vi "svm_save_model.vi"(8 "error in (no error)":errorcluster, 10 "Model":T1, 11 "Save path":path) -> (0 "error out":errorcluster)   [LabVIEW 2015]
uses:
  Controls/svm_model.ctl
  Controls/svm_parameter.ctl
  Controls/svm_type.ctl
  Controls/svm_kernel_type.ctl
  Controls/svm_node.ctl
  bin/LabVIEW-libsvm.so
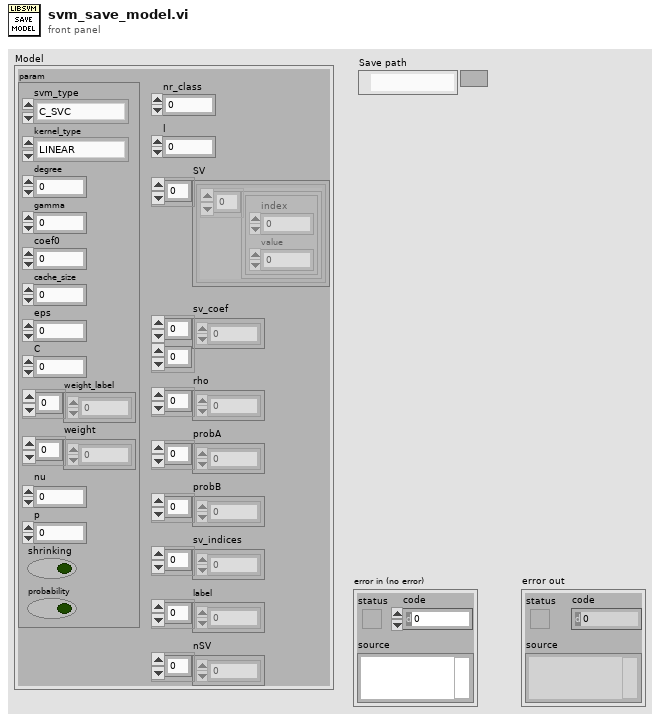
[diagram p1: front panel]
types:
  T1 = typedef "svm_model.ctl" = cluster{"param":T2, "nr_class":i32, "l":i32, "SV":cluster{"Array":T5[]}[], "sv_coef":dbl[][], "rho":dbl[], "probA":dbl[], "probB":dbl[], "sv_indices":i32[], "label":i32[], "nSV":i32[]}
  T2 = typedef "svm_parameter.ctl" = cluster{"svm_type":T3, "kernel_type":T4, "degree":i32, "gamma":dbl, "coef0":dbl, "cache_size":dbl, "eps":dbl, "C":dbl, "weight_label":i32[], "weight":dbl[], "nu":dbl, "p":dbl, "shrinking":bool, "probability":bool}
  T3 = typedef "svm_type.ctl" = enum32{"C_SVC", "NU_SVC", "ONE_CLASS", "EPSILON_SVR", "NU_SVR"}
  T4 = typedef "svm_kernel_type.ctl" = enum32{"LINEAR", "POLY", "RBF", "SIGMOID", "PRECOMPUTED"}
  T5 = typedef "svm_node.ctl" = cluster{"index":i32, "value":dbl}
  T6 = typedef "svm_model_padded.ctl" = cluster{"param":T2, "nr_class":i32, "l":i32, "SV":cluster{"Array":T7[]}[], "sv_coef":dbl[][], "rho":dbl[], "probA":dbl[], "probB":dbl[], "sv_indices":i32[], "label":i32[], "nSV":i32[]}
  T7 = typedef "svm_node_padded.ctl" = cluster{"index":i32, "padding":i32, "value":dbl}
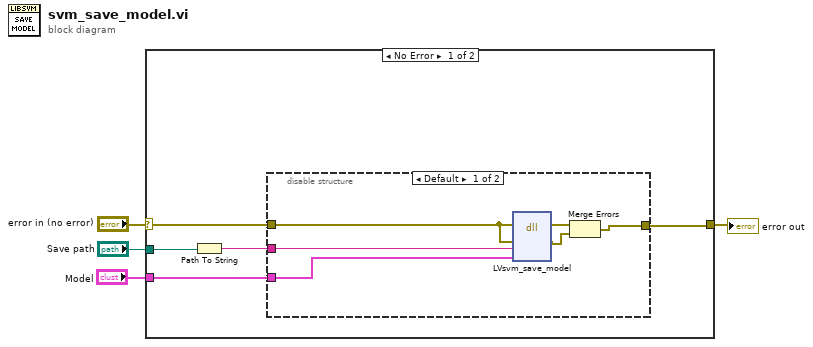
[diagram p0: block diagram]
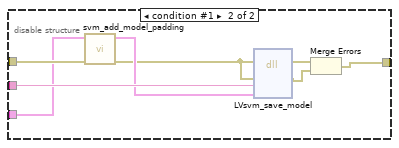
[diagram p2: hidden frame]
diagram:
  n1 = case shown="No Error" "error in (no error)" {
    selector: "error in (no error)" -> [w7 w24]
    tunnel: [w6 w24] -> w4
    tunnel: "Save path" -> [w9 _]
    tunnel: "Model" -> [w5 _]
    frame No Error {
      n2 = Path To String(path=w9) -> (string=w8:string)
      n3 = disable-structure shown="Default" {
        disable-tunnel: w8 -> [w15 w23]
        disable-tunnel: w7 -> [w10 w19]
        disable-tunnel: [w12 w20] -> w6
        disable-tunnel: w5 -> [w11 w18]
        frame condition #0 (active) {
          n4 = dll-call lib="home/os/dev/LabVIEW-libsvm/LabVIEW/bin/LabVIEW-libsvm.*" fn="LVsvm_save_model"(error in=w10, "lvErr"=w10, "path_in"=w15, "model_in"=w11) -> (error out=w14:errorcluster, "lvErr"=w13:errorcluster)  [unwired: 5 in, 1 out]
          n5 = Merge Errors(w14, w13) -> (w12:errorcluster)
        }
        frame condition #1 {
          n6 = call "svm_add_model_padding.vi"("error in (no error)"=w19, "Model"=w18) -> ("error out"=w16:errorcluster, "Padded model"=w17:T6)  [unwired: 8 in]
          n7 = dll-call lib="home/os/dev/LabVIEW-libsvm/LabVIEW/bin/LabVIEW-libsvm.*" fn="LVsvm_save_model"(error in=w16, "lvErr"=w16, "path_in"=w23, "model_in"=w17) -> (error out=w22:errorcluster, "lvErr"=w21:errorcluster)  [unwired: 5 in, 1 out]
          n8 = Merge Errors(w22, w21) -> (w20:errorcluster)
        }
      }
    }
    frame Error {
    }
  }
  "error out" <- w4
